vi "tryInsertToArr2D.vi"() -> ()   [LabVIEW 2010]
panel:
  in  "String":string
  in  "col":i32
  in  "row":i32
  in  "Table Control":string[][](table)
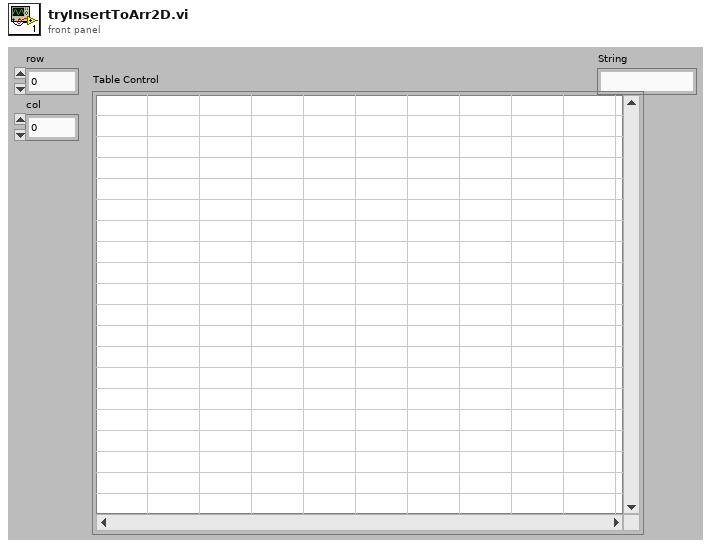
[diagram p1: front panel]
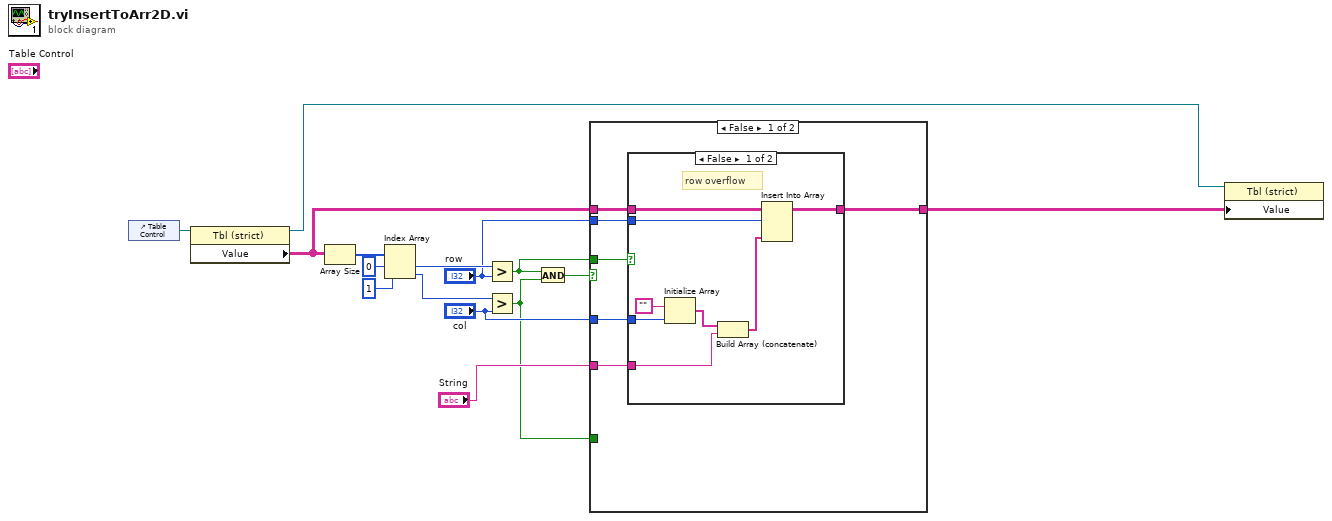
[diagram p0: block diagram]
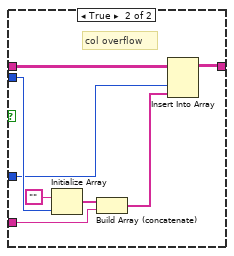
[diagram p2: hidden frame]
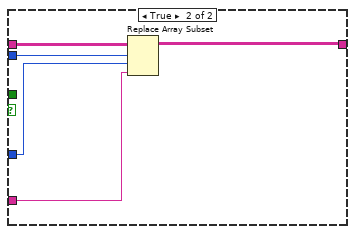
[diagram p3: hidden frame]
diagram:
  n1 = control-ref of="Table Control"() -> (w15:refnum<vi>)
  n2 = property class="Tbl (strict)"(reference=w15) -> (reference out=w6:refnum<vi>, "Value"=w9:string[][])  [unwired: 1 in, 1 out]
  n3 = Array Size(array=w9) -> (size(s)=w14:i32[])
  n4 = Index Array(array=w14, index #1=0 ("index"), index #2=1 ("index")) -> (element #1=w5:i32, element #2=w11:i32)
  n5 = Greater?(x=w5, y="row") -> (0:w3:bool)
  n6 = Greater?(x=w11, y="col") -> (0:w1:bool)
  n7 = And(x=w3, y=w1) -> (x .and. y?=w10:bool)
  n8 = case shown="False" w10 {
    tunnel: w9 -> [w18 w42]
    tunnel: "col" -> [w20 w40]
    tunnel: [w16 w39] -> w7
    tunnel: "row" -> [w17 w41]
    tunnel: w3 -> [w21 _]
    tunnel: "String" -> [w19 w38]
    tunnel: w1 -> [_ _]
    frame False {
      n9 = case shown="False" w21 {
        tunnel: w20 -> [w25 w30]
        tunnel: w19 -> [w23 w32]
        tunnel: w18 -> [w29 w37]
        tunnel: w17 -> [w27 w34]
        tunnel: [w28 w36] -> w16
        frame False {
          # "row overflow"
          n10 = Initialize Array("", w25) -> (w24:string[])
          n11 = Build Array (concatenate)(w24, w23) -> (w22:string[])
          n12 = Insert Into Array(array=w29, index (row)=w27, new element=w22) -> (w28:string[][])  [unwired: 1 in]
        }
        frame True {
          # "col overflow"
          n13 = Initialize Array("", w34) -> (w33:string[])
          n14 = Build Array (concatenate)(w33, w32) -> (w31:string[])
          n15 = Insert Into Array(array=w37, index (col)=w30, new element=w31) -> (w36:string[][])  [unwired: 1 in]
        }
      }
    }
    frame True {
      n16 = Replace Array Subset(array=w42, new element=w38, index (row)=w41, index (col)=w40) -> (w39:string[][])
    }
  }
  n17 = property class="Tbl (strict)"(reference=w6, "Value"=w7) -> ()  [unwired: 1 in, 2 out]
